vi "API_DB.GetAllLocationsInStocker.vi"(0 "Database in":refnum<class "Database.lvclass">, 1 "Wait (F)":bool, 5 "Table":string, 7 "InventoryRecord.Stocker":T1 items=["Main", "Exp1", "Exp2"], 11 "error in (no error)":errorcluster, 12 "Timeout (ms)":u32) -> (4 "Database out":refnum<class "Database.lvclass">, 6 "Slot":string, 15 "error out":errorcluster)   [LabVIEW 2022 SP3]
doc: "Developed by Kevin Thompson\nkevin@thompsonengineering.net\n\nCopyright 2018\nThompson Engineering, LLC"
uses:
  Database.lvclass
  DataTypes/AsynCmd_Temp01--enum.ctl
  DataTypes/GenericQuery--Cluster.ctl
  DataTypes/SQLQuery--Enum.ctl
  Database.lvclass/Database.ctl
  DataTypes/Stocker--Enum.ctl
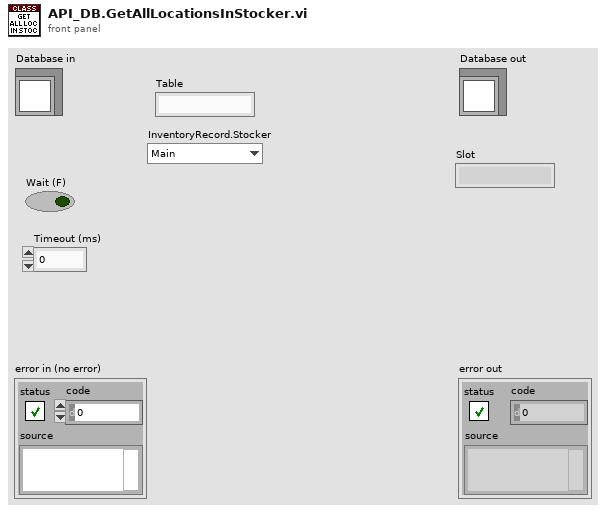
[diagram p1: front panel]
types:
  T1 = typedef "Stocker--Enum.ctl" = u16
  T2 = typedef "SQLQuery--Enum.ctl" = enum16{"GetAllMaterials", "GetAllColors"}
  T3 = typedef "GenericQuery--Cluster.ctl" = cluster{"Query":T2, "Table":string}
  T4 = typedef "Database.lvclass/AsynCmd_Temp01--enum.ctl" = enum16{"DB.DeleteRecord", "DB.UpdateRecord", "DB.InsertRecord", "DB.SelectRecord", "DB.ExecuteSQLCommand", "DB.FindFirstSlot", "DB.GenericSQLQuery"}
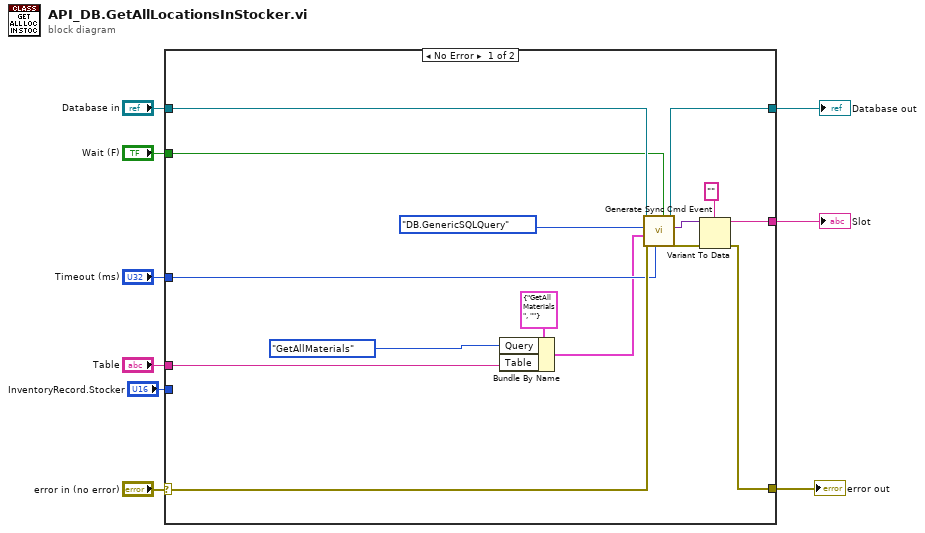
[diagram p0: block diagram]
diagram:
  n1 = case shown="No Error" "error in (no error)" {
    selector: "error in (no error)" -> [w22 w26]
    tunnel: [w17 w26] -> w8
    tunnel: [w23 w25] -> w6
    tunnel: "Database in" -> [w24 w25]
    tunnel: [w19 _] -> w3
    tunnel: "Wait (F)" -> [w16 _]
    tunnel: "Timeout (ms)" -> [w15 _]
    tunnel: "Table" -> [w10 _]
    tunnel: "InventoryRecord.Stocker" -> [_ _]
    frame No Error {
      n2 = Bundle By Name(cluster=T3 {"Query"=enum."GetAllMaterials", "Table"=""}, "Query"=SQLQuery--Enum."GetAllMaterials", "Table"=w10) -> (w11:T3)
      n3 = call "Generate Sync Cmd Event.vi"("Wait (F)"=w16, "Timeout (ms)"=w15, "error in (no error)"=w22, "vData"=w11, "AsyncCmd"=AsynCmd_Temp01--enum."DB.GenericSQLQuery", "Database in"=w24) -> ("error out"=w18:errorcluster, "Return Value"=w20:variant, "Database out"=w23:refnum<class "Database.lvclass">)  [unwired: 3 in]
      n4 = Variant To Data(error in=w18, type="", Variant=w20) -> (data=w19:string, error out=w17:errorcluster)
    }
    frame Error {
    }
  }
  "error out" <- w8
  "Database out" <- w6
  "Slot" <- w3
